vi "Self-Test.vi"(8 "error in (no error)":errorcluster, 11 "VISA resource name":refnum<visa-resource-name>) -> (0 "error out":errorcluster, 1 "Self-Test Result Message":string, 2 "Self-Test Result Code":i32, 3 "VISA resource name out":refnum<visa-resource-name>)   [LabVIEW 2021, in "Yokogawa WT1800 Series.lvlib"]
doc: "Runs the instrument's self-test routine and returns the test results."
uses:
  <instrlib>/Yokogawa WT1800 Series/Yokogawa WT1800 Series.lvlib
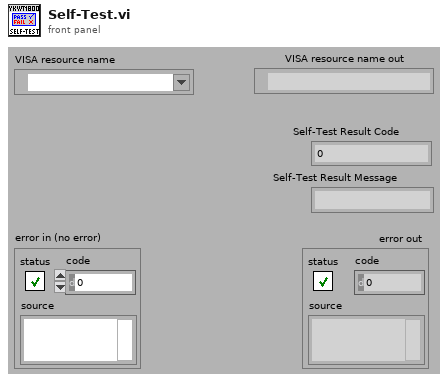
[diagram p1: front panel]
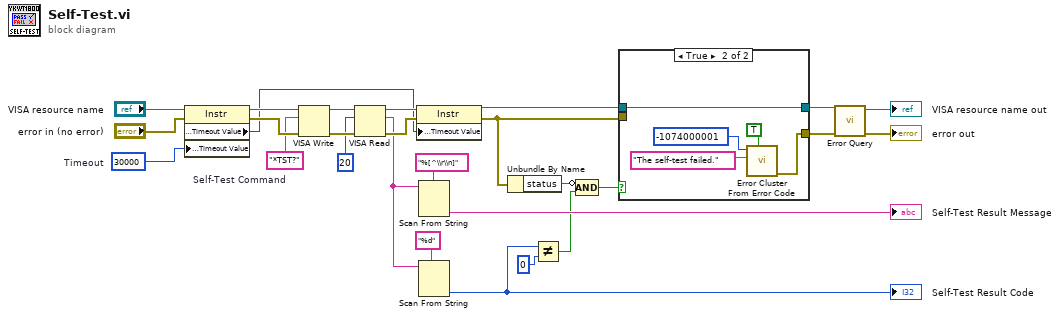
[diagram p0: block diagram]
diagram:
  w15 = u32 30000  # Timeout
  w11 = "*TST?"  # Self-Test Command
  n1 = property class="Instr"(reference="VISA resource name", error in="error in (no error)", "General Settings:Timeout Value"=w15) -> (reference out=w13:refnum<visa-resource-name>, error out=w14:errorcluster, "General Settings:Timeout Value"=w12:u32)
  n2 = VISA Write(VISA resource name=w13, write buffer=w11, error in (no error)=w14) -> (VISA resource name out=w24:refnum<visa-resource-name>, error out=w23:errorcluster)  [unwired: 1 out]
  n3 = VISA Read(VISA resource name=w24, byte count=u32 20 ("byte count (20)"), error in (no error)=w23) -> (VISA resource name out=w26:refnum<visa-resource-name>, read buffer=w19:string, error out=w25:errorcluster)  [unwired: 1 out]
  n4 = property class="Instr"(reference=w26, error in=w25, "General Settings:Timeout Value"=w12) -> (reference out=w10:refnum<visa-resource-name>, error out=w9:errorcluster)
  n5 = Scan From String(format string="%[^\\r\\n]" ("Format String"), input string=w19) -> (output 1=→"Self-Test Result Message":string)  [unwired: 3 in, 3 out]
  n6 = Scan From String(format string="%d", input string=w19) -> (output 1=w2:i32)  [unwired: 3 in, 3 out]
  "Self-Test Result Code" <- w2
  n7 = Unbundle By Name(w9) -> ("status"=w5:bool)
  n8 = Not Equal?(x=w2, y=0) -> (x != y?=w6:bool)
  n9 = Compound Arithmetic op=AND(invert w5, w6) -> (w4:bool)
  n10 = case shown="True" w4 {
    tunnel: w10 -> [w29 w34]
    tunnel: w9 -> [w28 _]
    tunnel: [w28 w30] -> w8
    tunnel: [w29 w34] -> w7
    frame False {
    }
    frame True {
      n11 = call <vilib>:"Error Cluster From Error Code.vi"("show call chain? (False)"=TRUE, "error message (\"\")"="The self-test failed." ("Source (VI Name)"), "error code (0)"=-1074000001 ("Code")) -> ("error out"=w30:errorcluster)  [unwired: 6 in]
    }
  }
  n12 = call <instrlib>:"Error Query.vi"("error in (no error)"=w8, "VISA resource name"=w7) -> ("error out"=→"error out":errorcluster, "VISA resource name out"=→"VISA resource name out":refnum<visa-resource-name>)  [unwired: 6 in, 2 out]
